vi "Read_Monitor_OPCDA_Tags_LabVIEW.vi"() -> ()   [LabVIEW 2024]
panel:
  out "Triangle.PsFloat1":dbl
  out "Sinusoid.PsFloat1":dbl
  out "Triangle.PsInteger1":dbl
  out "Random.PsFloat1":dbl
  out "SawTooth.PsFloat1":dbl
  out "Sinusoid.PsInteger1":dbl
  out "SawTooth.PsInteger1":dbl
  out "Random.PsInteger1":dbl
  out "Error Connecting OPCDA Server":bool
  out "Error Reading Data from OPCDA Server":bool
  out "Recent Data Read Time Stamp":timestamp format="%<%x %.3X>T"
  in  "Interval (ms)":dbl=500.0
  out "OPCDA Close Connection Error":errorcluster
  out "Timeout from OPCDA Server":bool
  in  "Stop Button":bool
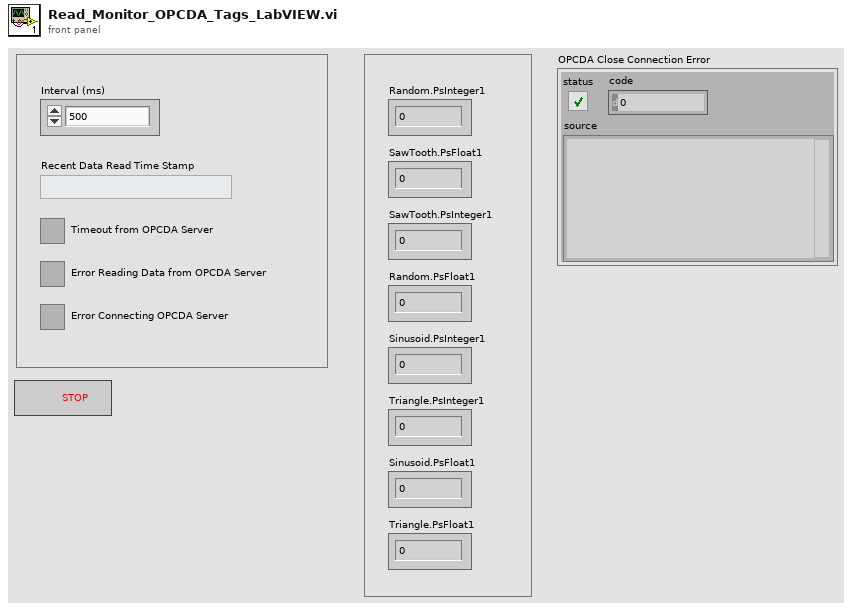
[diagram p1: front panel]
types:
  T1 = enum16{"Read", "Write", "ReadWrite", "BufferedRead", "BufferedReadWrite"}
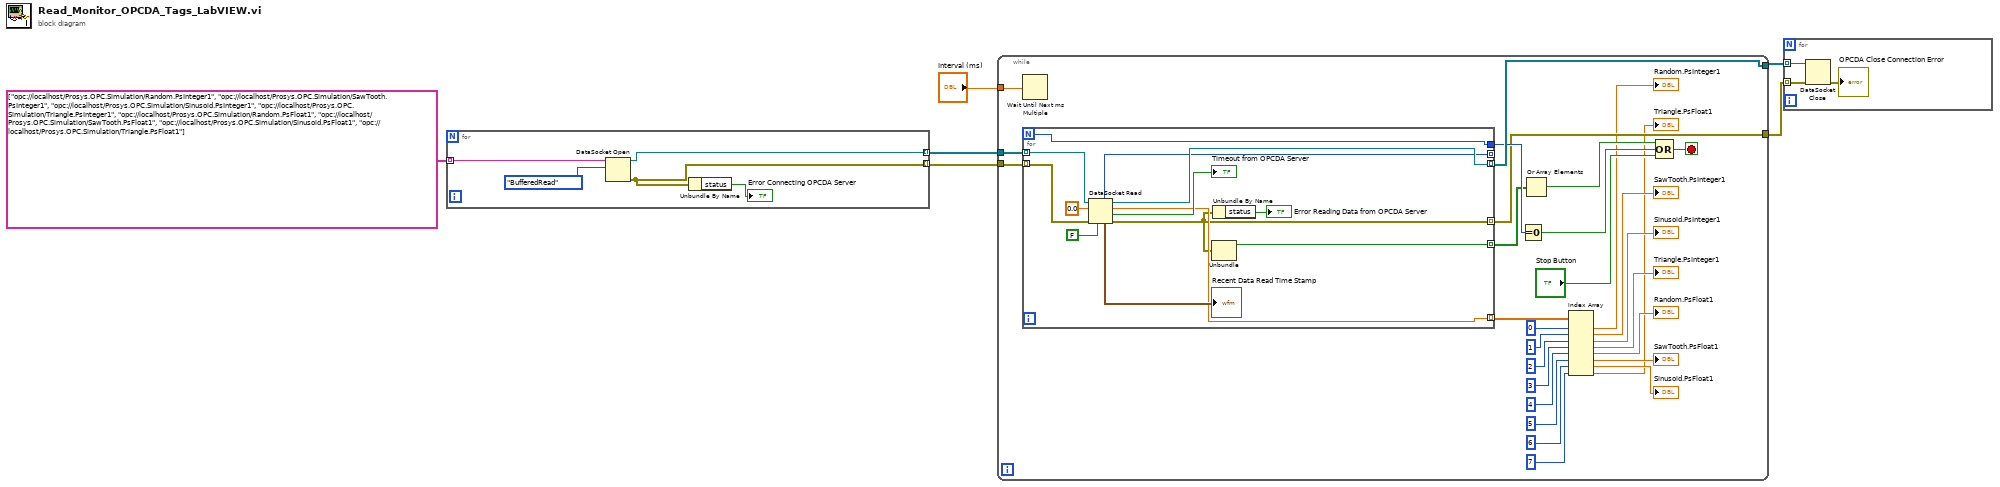
[diagram p0: block diagram]
diagram:
  n1 = for {
    tunnel: [w11] -> w3 mode=indexing
    tunnel: [w7] -> w2 mode=indexing
    tunnel: string[] ["opc://localhost/Prosys.OPC.Simulation/Random.PsInteger1", "opc://localhost/Prosys.OPC.Simulation/SawTooth.PsInteger1", "opc://localhost/Prosys.OPC.Simulation/Sinusoid.PsInteger1", "opc://localhost/Prosys.OPC.Simulation/Triangle.PsInteger1", "opc://localhost/Prosys.OPC.Simulation/Random.PsFloat1", "opc://localhost/Prosys.OPC.Simulation/SawTooth.PsFloat1", "opc://localhost/Prosys.OPC.Simulation/Sinusoid.PsFloat1", "opc://localhost/Prosys.OPC.Simulation/Triangle.PsFloat1"] ("all rows") -> [w9] mode=indexing
    n2 = DataSocket Open(10:T1."BufferedRead" ("mode"), 11:w9) -> (0:w7:errorcluster, 3:w11:refnum<k13>)  [unwired: 1 in, 1 out]
    n3 = Unbundle By Name(w7) -> ("status"=→"Error Connecting OPCDA Server":bool)
  }
  n4 = while {
    tunnel: [w37] -> w5
    tunnel: [w39] -> w6
    tunnel: w3 -> [w31]
    tunnel: w2 -> [w30]
    tunnel: "Interval (ms)" -> [w12]
    stop <- w32 stop-if-true
    n5 = Wait Until Next ms Multiple(millisecond multiple=w12) -> ()  [unwired: 1 out]
    n6 = for {
      N -> [w51]
      tunnel: w31 -> [w46] mode=indexing
      tunnel: [w52] -> w39 mode=indexing
      tunnel: [w51] -> w38
      tunnel: w30 -> [w50] mode=indexing
      tunnel: [w40] -> w37 mode=indexing
      tunnel: [w44] -> w13 mode=indexing
      tunnel: [w43] -> _ mode=indexing
      tunnel: [w42] -> w35 mode=indexing
      n7 = DataSocket Read(6:FALSE ("wait for updated value (T)"), 8:w50, 10:0.0, 11:w46) -> (0:w40:errorcluster, 1:→"Timeout from OPCDA Server":bool, 2:w44:dbl, 3:w52:refnum<k13>, 4:→"Recent Data Read Time Stamp":timestamp, 5:w43:u64)  [unwired: 2 out]
      n8 = Unbundle "Unbundle"(w40) -> ("status"=w42:bool)  [unwired: 2 out]
      n9 = Unbundle By Name(w40) -> ("status"=→"Error Reading Data from OPCDA Server":bool)
    }
    n10 = Equal To 0?(x=w38) -> (x = 0?=w36:bool)
    n11 = Or Array Elements(Boolean array=w35) -> (logical OR=w34:bool)
    n12 = Index Array(array=w13, index #1=0 ("index"), index #2=1 ("index"), index #3=2 ("index"), index #4=3 ("index"), index #5=4 ("index"), index #6=5 ("index"), index #7=6 ("index"), index #8=7 ("index")) -> (element #1=→"Random.PsInteger1":dbl, element #2=→"SawTooth.PsInteger1":dbl, element #3=→"Sinusoid.PsInteger1":dbl, element #4=→"Triangle.PsInteger1":dbl, element #5=→"Random.PsFloat1":dbl, element #6=→"SawTooth.PsFloat1":dbl, element #7=→"Sinusoid.PsFloat1":dbl, element #8=→"Triangle.PsFloat1":dbl)
    n13 = Compound Arithmetic op=OR(w34, w36, "Stop Button") -> (w32:bool)
  }
  n14 = for {
    tunnel: w6 -> [w55] mode=indexing
    tunnel: w5 -> [w54] mode=indexing
    n15 = DataSocket Close(8:w54, 11:w55) -> (0:→"OPCDA Close Connection Error":errorcluster)  [unwired: 2 out]
  }
